vi "StringCaseStructure.vi"() -> ()   [LabVIEW 2019]
panel:
  in  "String":string
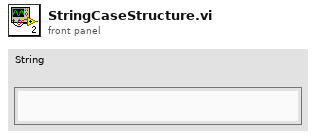
[diagram p1: front panel]
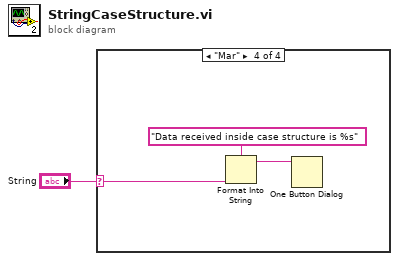
[diagram p0: block diagram]
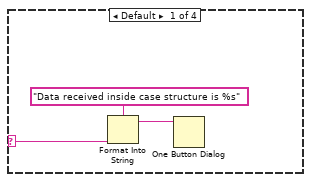
[diagram p2: hidden frame]
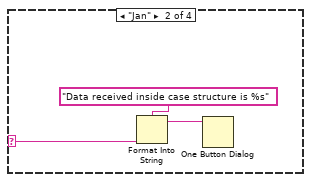
[diagram p3: hidden frame]
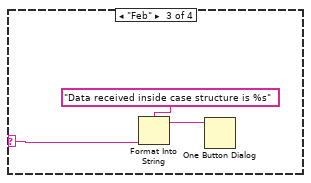
[diagram p4: hidden frame]
diagram:
  n1 = case shown="\"Mar\"" "String" {
    selector: "String" -> [w4 w5 w8 w11]
    frame Default {
      n2 = Format Into String(format string="Data received inside case structure is %s", w4) -> (resulting string=w2:string)  [unwired: 2 in, 1 out]
      n3 = One Button Dialog(message=w2) -> ()  [unwired: 1 in, 1 out]
    }
    frame "Jan" {
      n4 = Format Into String(format string="Data received inside case structure is %s", w5) -> (resulting string=w7:string)  [unwired: 2 in, 1 out]
      n5 = One Button Dialog(message=w7) -> ()  [unwired: 1 in, 1 out]
    }
    frame "Feb" {
      n6 = Format Into String(format string="Data received inside case structure is %s", w8) -> (resulting string=w10:string)  [unwired: 2 in, 1 out]
      n7 = One Button Dialog(message=w10) -> ()  [unwired: 1 in, 1 out]
    }
    frame "Mar" {
      n8 = Format Into String(format string="Data received inside case structure is %s", w11) -> (resulting string=w13:string)  [unwired: 2 in, 1 out]
      n9 = One Button Dialog(message=w13) -> ()  [unwired: 1 in, 1 out]
    }
  }
